vi "Out_S2F42.vi"(8 "error in (no error)":errorcluster, 10 "S2F42":T1, 11 "S2 Message Class in":refnum<class "S2 Message Class.lvclass">) -> (0 "error out":errorcluster, 3 "S2 Message Class out":refnum<class "S2 Message Class.lvclass">)   [LabVIEW 2020, in "SECS Communication.lvlib" / "S2 Message Class.lvclass"]
uses:
  S2 Message Class.lvclass
  D:/Dropbox/SECS/SECS_GEM v1.0.6/Com/SECS Communication/SECS-II Class/SECS-II Class.lvclass
  S2F42.ctl
  SECS-II Class/Data Message_List.vi
  SECS-II Class/Data Message_Binary.vi
  SECS-II Class/Data Message_ASCII.vi
  SECS-II Class/SECS-II Class.lvclass
  D:/Dropbox/SECS/SECS_GEM v1.0.6/Com/SECS Communication/S2 Message Class/S2 Message Class.lvclass
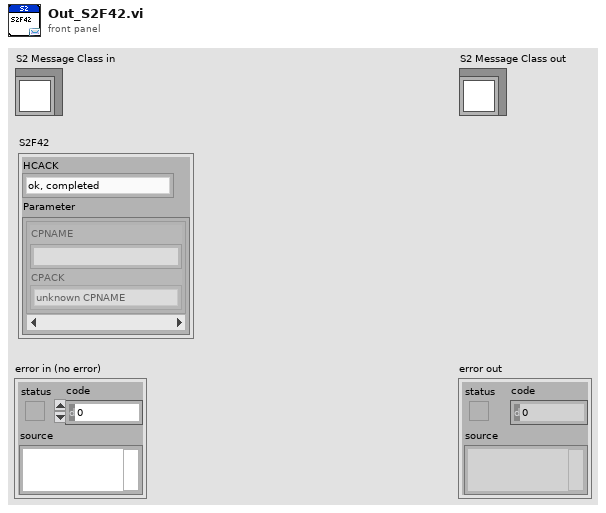
[diagram p1: front panel]
types:
  T1 = typedef "SECS Communication.lvlib/S2 Message Class.lvclass/S2F42.ctl" = cluster{"HCACK":enum8{"ok, completed", "invalid command", "cannot do now", "parameter error", "initiated for asynchronous completion", "rejected, already in desired condition", "invalid object"}, "Parameter ":cluster{"CPNAME":string, "CPACK":enum8{"unknown CPNAME", "illegal value for CPVAL", "illegal format for CPVAL"}}[]}
  T2 = enum8{"ok, completed", "invalid command", "cannot do now", "parameter error", "initiated for asynchronous completion", "rejected, already in desired condition", "invalid object"}
  T3 = cluster{"CPNAME":string, "CPACK":enum8{"unknown CPNAME", "illegal value for CPVAL", "illegal format for CPVAL"}}[]
  T4 = enum8{"unknown CPNAME", "illegal value for CPVAL", "illegal format for CPVAL"}
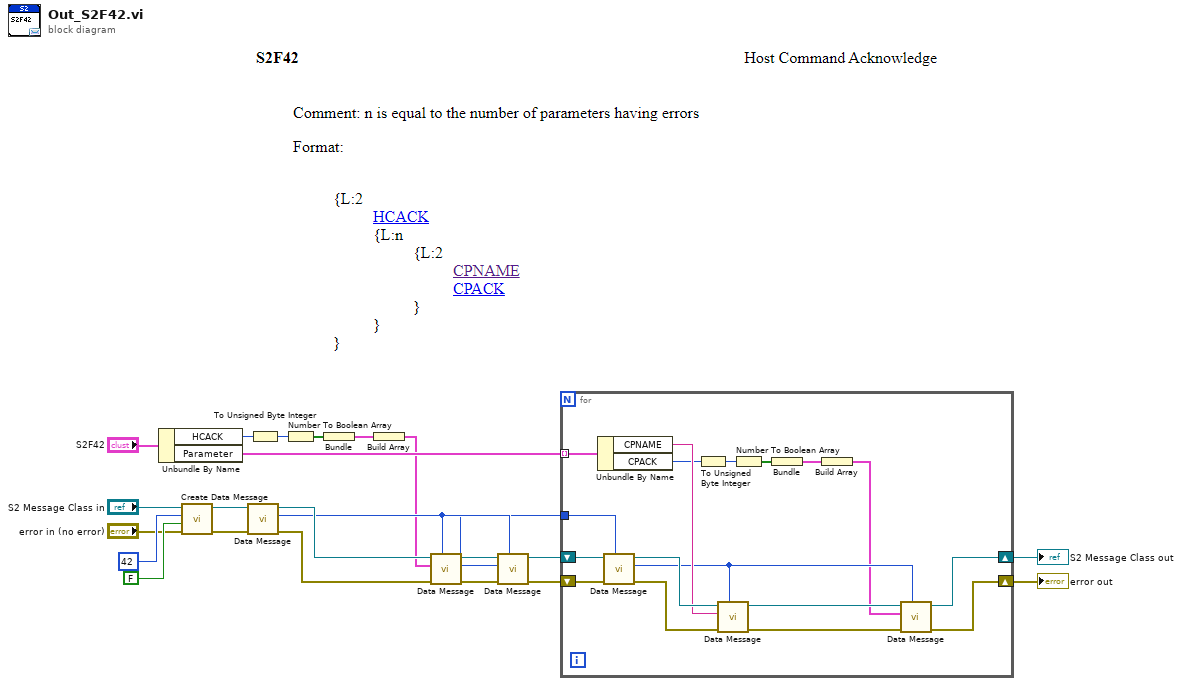
[diagram p0: block diagram]
diagram:
  n1 = Unbundle By Name("S2F42") -> ("HCACK"=w7:T2, "Parameter"=w11:T3)
  n2 = call "Create Data Message.vi"("error in (no error)"="error in (no error)", "W-Bit"=FALSE, "Function"=u8 42, "SECS-II Class in"="S2 Message Class in") -> ("error out"=w9:errorcluster, "SECS-II Class out"=w10:refnum<class "S2 Message Class.lvclass">)  [unwired: 6 in]
  n3 = call-poly "Data Message.vi"("error in"=w9, "SECS-II Class in"=w10) -> ("error out"=w18:errorcluster, "Index"=w15:i32, "SECS-II Class out"=w19:refnum<class "S2 Message Class.lvclass">)  [unwired: 7 in]
  n4 = To Unsigned Byte Integer(number=w7) -> (unsigned 8bit integer=w6:u8)
  n5 = Number To Boolean Array(number=w6) -> (Boolean array=w5:bool[])
  n6 = Bundle("Boolean array"=w5) -> (w4:cluster{"Boolean array":bool[]})  [unwired: 1 in]
  n7 = Build Array(w4) -> (w3:cluster{"Boolean array":bool[]}[])
  n8 = call-poly "Data Message.vi"("Parent Index"=w15, "error in"=w18, "Data Cluster"=w3, "SECS-II Class in"=w19) -> ("error out"=w16:errorcluster, "SECS-II Class out"=w17:refnum<class "S2 Message Class.lvclass">)  [unwired: 6 in]
  n9 = call-poly "Data Message.vi"("Parent Index"=w15, "error in"=w16, "SECS-II Class in"=w17) -> ("error out"=w13:errorcluster, "Index"=w12:i32, "SECS-II Class out"=w14:refnum<class "S2 Message Class.lvclass">)  [unwired: 6 in]
  n10 = for {
    shift-right: [w29] -> w1
    shift-left: w13 -> [w40]
    shift-right: [w30] -> w2
    shift-left: w14 -> [w39]
    tunnel: w12 -> [w38]
    tunnel: w11 -> [w35] mode=indexing
    n11 = Unbundle By Name(w35) -> ("CPNAME"=w34:string, "CPACK"=w28:T4)
    n12 = call-poly "Data Message.vi"("Parent Index"=w38, "error in"=w40, "SECS-II Class in"=w39) -> ("error out"=w37:errorcluster, "Index"=w31:i32, "SECS-II Class out"=w36:refnum<class "S2 Message Class.lvclass">)  [unwired: 6 in]
    n13 = To Unsigned Byte Integer(number=w28) -> (unsigned 8bit integer=w27:u8)
    n14 = call-poly "Data Message.vi"("Parent Index"=w31, "error in"=w37, "Data"=w34, "SECS-II Class in"=w36) -> ("error out"=w32:errorcluster, "SECS-II Class out"=w33:refnum<class "S2 Message Class.lvclass">)  [unwired: 6 in]
    n15 = Number To Boolean Array(number=w27) -> (Boolean array=w26:bool[])
    n16 = Bundle("Boolean array"=w26) -> (w25:cluster{"Boolean array":bool[]})  [unwired: 1 in]
    n17 = Build Array(w25) -> (w24:cluster{"Boolean array":bool[]}[])
    n18 = call-poly "Data Message.vi"("Parent Index"=w31, "error in"=w32, "Data Cluster"=w24, "SECS-II Class in"=w33) -> ("error out"=w29:errorcluster, "SECS-II Class out"=w30:refnum<class "S2 Message Class.lvclass">)  [unwired: 6 in]
  }
  "error out" <- w1
  "S2 Message Class out" <- w2
